vi "AIRE ACONDICIONADO.vi"() -> ()   [LabVIEW 2017]
panel:
  out "Temperatura":i64(slide) scale=0.0..50.0
  in  "Iniciar el Proceso":bool
  in  "Ingrese Temperatura Deseada":i64
  in  "Ingrese temperatura Ambiente":i64
  # "El usuario ingresa la temperatura ambiente y deseada, luego presiona el botón Iniciar Proceso. \nLa temperatura sube o baja depende de los valores ingresados por el usuario. \nEj Si la temperatura ambiente es de10° y la temperatura deseada es de 21°, el termómetro iniciará el 10 \ne irá subiendo 1 grado a la vez cada 500 milisegundos, hasta llegar a 21.\n\nEl programa termina cuanto el usuario presione el botón Apagar el Aire. \nEl botón puede ser sustituido por un mensaje emergente al usuario"
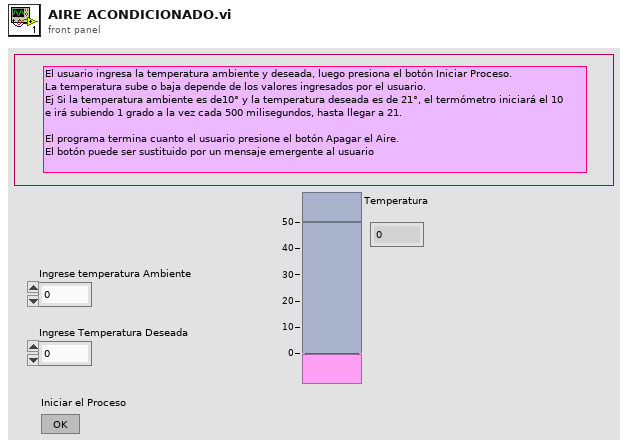
[diagram p1: front panel]
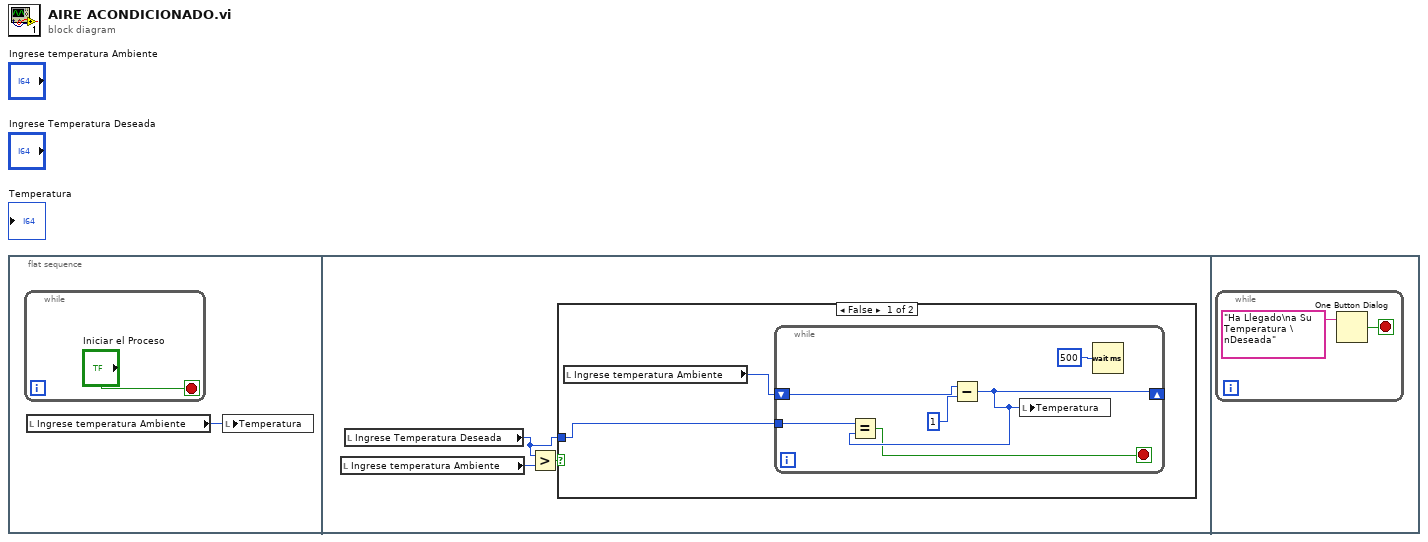
[diagram p0: block diagram]
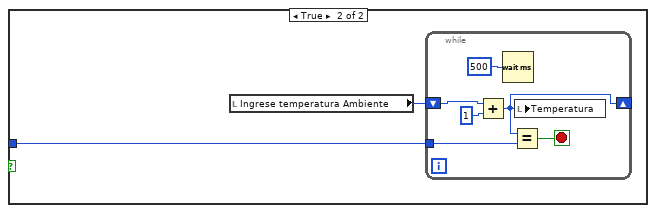
[diagram p2: hidden frame]
diagram:
  n1 = flat-sequence {
    frame #0 {
      n2 = while {
        stop <- "Iniciar el Proceso" stop-if-true
      }
      n3 = local read "Ingrese temperatura Ambiente"() -> (w1:i64)
      n4 = local write "Temperatura"(w1) -> ()
    }
    frame #1 {
      n5 = local read "Ingrese temperatura Ambiente"() -> (w5:i64)
      n6 = local read "Ingrese Temperatura Deseada"() -> (w3:i64)
      n7 = Greater?(x=w3, y=w5) -> (0:w4:bool)
      n8 = case shown="False" w4 {
        tunnel: w3 -> [w6 w14]
        frame False {
          n9 = local read "Ingrese temperatura Ambiente"() -> (w7:i64)
          n10 = while {
            shift-right: [w9] -> _
            shift-left: w7 -> [w12]
            tunnel: w6 -> [w10]
            stop <- w8 stop-if-true
            n11 = Subtract(x=w12, y=i64 1) -> (x-y=w9:i64)
            n12 = Equal?(x=w10, y=w9) -> (x = y?=w8:bool)
            n13 = local write "Temperatura"(w9) -> ()
            n14 = Wait (ms)(milliseconds to wait=u32 500) -> ()  [unwired: 1 out]
          }
        }
        frame True {
          n15 = local read "Ingrese temperatura Ambiente"() -> (w15:i64)
          n16 = while {
            shift-right: [w18] -> _
            shift-left: w15 -> [w19]
            tunnel: w14 -> [w17]
            stop <- w16 stop-if-true
            n17 = Add(x=w19, y=i64 1) -> (x+y=w18:i64)
            n18 = Wait (ms)(milliseconds to wait=u32 500) -> ()  [unwired: 1 out]
            n19 = Equal?(x=w18, y=w17) -> (x = y?=w16:bool)
            n20 = local write "Temperatura"(w18) -> ()
          }
        }
      }
    }
    frame #2 {
      n21 = while {
        stop <- w22 stop-if-true
        n22 = One Button Dialog(message="Ha Llegado\na Su Temperatura \nDeseada") -> (true=w22:bool)  [unwired: 1 in]
      }
    }
  }
